vi "macro_LTV_DiffDriveCtrl_Traj_Sample_Execute.vi"() -> ()   [LabVIEW 2019, in "Trajectory_Library.lvlib"]
uses:
  Trajectory_Library.lvlib
  TypeDef/POSE2D.ctl
  TypeDef/TRANSLATION2D.ctl
  TypeDef/ROTATION2D.ctl
  TypeDef/TRAJ_STATE.ctl
  Enum/DCMOTOR_TYPES_ENUM.ctl
  Enum/DIFF_DRIVE_ToughBoxMini_GearChoice_ENUM.ctl
  LinearSystemId_CreateDriveTrainVelocitySystem.vi
  DCMotor_PickMotor_OLD.vi
  LinearSystem_New.vi
  MatBuilder_Create.vi
  MatBuilder_Fill.vi
  MatrixHelper_Zero.vi
  DCMotor_GetCIM.vi
  DCMotor_GetAndymark9015.vi
  DCMotor_GetAndymarkRs775_125.vi
  DCMotor_GetBag.vi
  DCMotor_GetBanebotsRs550.vi
  DCMotor_GetBanebotsRs775.vi
  DCMotor_GetFalcon500.vi
  DCMotor_GetMiniCIM.vi
  DCMotor_GetNEO.vi
  DCMotor_GetNEO550.vi
  DCMotor_GetRomiBuiltIn.vi
  DCMotor_GetVex775Pro.vi
  VI/DCMotor_GetAndymarkAM2235A.vi
  VI/DCMotor_GetAndymarkAM3493.vi
  MatrixHelper_CoerceSize.vi
  DCMotor_New.vi
  VI/Units_RotationsPerMinuteToRadiansPerSecond.vi
panel:
  in  "TRAJ_STATE":T1={"TimeSeconds"=0.0, "Velocity"=0.0, "Acceleration"=0.0, "POSE"={"TRANSLATION"={"X"=0.0, "Y"=0.0}, "ROTATION"={"VALUE"=0.0, "COS"=1.0, "SIN"=0.0}}, "Curvature"=0.0} {"POSE"."ROTATION"."SIN" format="%13.4f"; "POSE"."ROTATION"."COS" format="%13.4f"; "POSE"."ROTATION"."VALUE" format="%13.4f"; "POSE"."TRANSLATION"."Y" format="%14.3f"; "POSE"."TRANSLATION"."X" format="%14.3f"}
  in  "Right Velocity":dbl
  in  "Left Velocity":dbl
  out "Right Motor Dmd":dbl
  out "Left Motor Dmd":dbl
  in  "CurrentPose":T2={"TRANSLATION"={"X"=0.0, "Y"=0.0}, "ROTATION"={"VALUE"=0.0, "COS"=1.0, "SIN"=0.0}} {"ROTATION"."SIN" format="%13.4f"; "ROTATION"."COS" format="%13.4f"; "ROTATION"."VALUE" format="%13.4f"; "TRANSLATION"."Y" format="%14.3f"; "TRANSLATION"."X" format="%14.3f"}
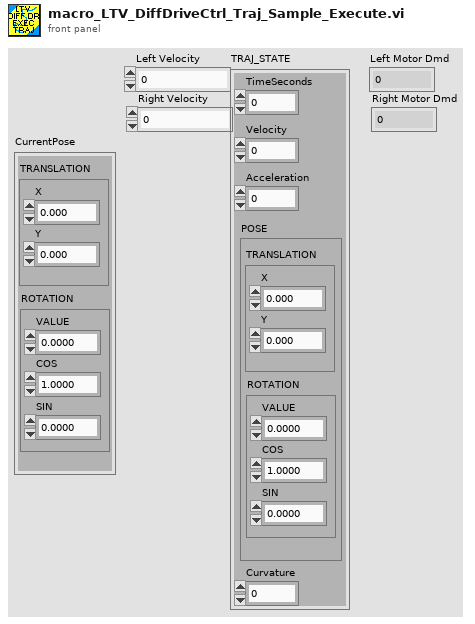
[diagram p1: front panel]
types:
  T1 = typedef "Trajectory_Library.lvlib/TRAJ_STATE.ctl" = cluster{"TimeSeconds":dbl, "Velocity":dbl, "Acceleration":dbl, "POSE":T2, "Curvature":dbl}
  T2 = typedef "Trajectory_Library.lvlib/POSE2D.ctl" = cluster{"TRANSLATION":T3, "ROTATION":T4}
  T3 = typedef "Trajectory_Library.lvlib/TRANSLATION2D.ctl" = cluster{"X":dbl, "Y":dbl}
  T4 = typedef "Trajectory_Library.lvlib/ROTATION2D.ctl" = cluster{"VALUE":dbl, "COS":dbl, "SIN":dbl}
  T5 = typedef "Trajectory_Library.lvlib/DIFF_DRIVE_ToughBoxMini_GearChoice_ENUM.ctl" = enum16{"Ratio_12_75", "Ratio_10_71", "Ratio_8_45", "Ratio_7_31", "Ratio_5_95"}
  T6 = typedef "Trajectory_Library.lvlib/DCMOTOR_TYPES_ENUM.ctl" = enum16{"CIM", "AndyMark 9015", "Andy Mark RS 775 125", "Bag", "BaneBots RS 550", "BaneBots RS 775", "Falcon 500", "Mini CIM", "NEO", "NEO 550", "Romi BuiltIn", "Vex 775 Pro", "Snow Blower AM 2235A", "Bosch Seat AM 3493"}
  T7 = typedef "Trajectory_Library.lvlib/LINEAR_SYSTEM.ctl" = cluster{"m_A":T8, "m_B":T8, "m_C":T8, "m_D":T8, "States":i32, "Inputs":i32, "Outputs":i32}
  T8 = typedef "NI_Matrix.lvlib/RealMatrix.ctl" = dbl[][]
  T9 = typedef "Trajectory_Library.lvlib/LTV_DIFF_DRIVE_CTRL_TOLERANCE.CTL" = cluster{"Max Heading Tolerance Rad":dbl, "Max X Tolerance M":dbl, "Max Y Tolerance M":dbl, "Max Left Vel Tol M/S":dbl, "Max Right Vel Tol M/S":dbl}
  T10 = typedef "Trajectory_Library.lvlib/LTV_DIFF_DRIVE_CTRL_CONTROL_PARAMS.CTL" = cluster{"Max left vel ctrl effort V":dbl, "Desired Heading Ctrl Tol Rad":dbl, "Desired Y Pos Meas Tol M":dbl, "Desired X Pos Ctrl Tol M":dbl, "Desired Left Vel Ctrl Tol M/S":dbl, "Desired Right Vel Ctrl Tol M/S":dbl, "Max right vel ctrl effort V":dbl}
  T11 = typedef "Trajectory_Library.lvlib/LTV_DIFF_DRIVE_CTRL_MODEL_PARAMS.CTL" = cluster{"Track Width":dbl, "Diff_Drive_Linear_System":T7, "LTV_DiffDriveCtrl_Control":T10, "LTV_DiffDriveCtrl_Tolerance":T9, "dT Sec":dbl}
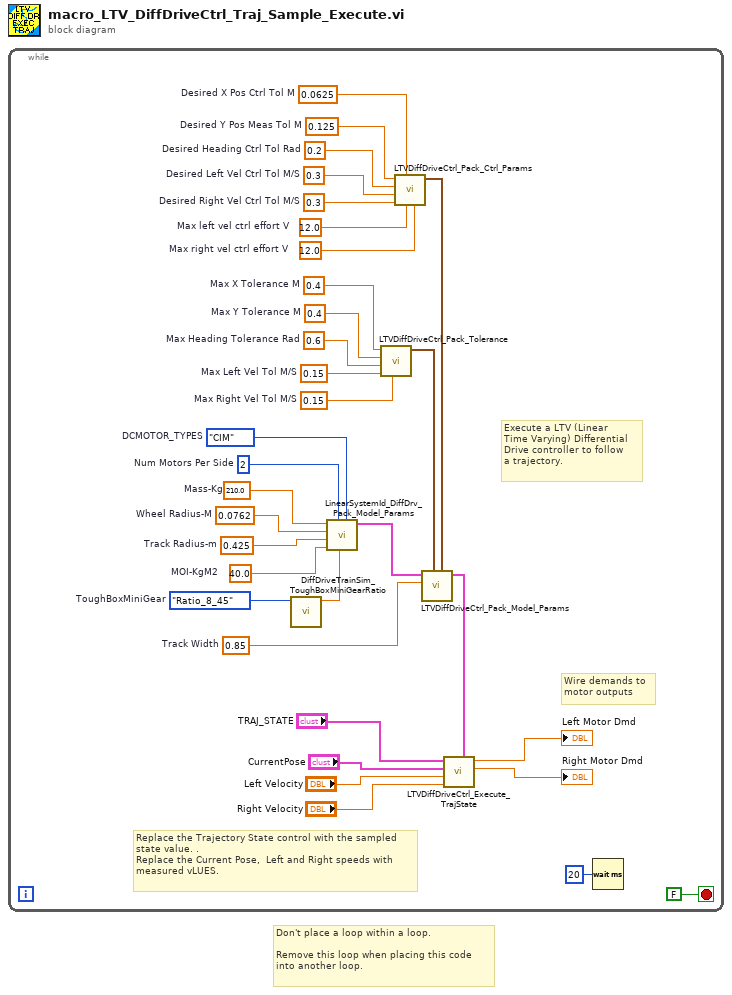
[diagram p0: block diagram]
diagram:
  # "Don't place a loop within a loop.\n \nRemove this loop when placing this code\ninto another loop."
  n1 = while {
    stop <- FALSE stop-if-true
    w6 = DIFF_DRIVE_ToughBoxMini_GearChoice_ENUM."Ratio_8_45"  # ToughBoxMiniGear
    w7 = 210.0  # Mass-Kg
    w8 = 0.0762  # Wheel Radius-M
    w9 = 0.425  # Track Radius-m
    w10 = 40.0  # MOI-KgM2
    w11 = 2  # Num Motors Per Side
    w12 = DCMOTOR_TYPES_ENUM."CIM"  # DCMOTOR_TYPES
    w14 = 0.4  # Max X Tolerance M
    w15 = 0.4  # Max Y Tolerance M
    w16 = 0.6  # Max Heading Tolerance Rad
    w17 = 0.15  # Max Left Vel Tol M/S
    w18 = 0.15  # Max Right Vel Tol M/S
    w19 = 0.125  # Desired Y Pos Meas Tol M
    w20 = 0.2  # Desired Heading Ctrl Tol Rad
    w21 = 0.3  # Desired Left Vel Ctrl Tol M/S
    w22 = 0.3  # Desired Right Vel Ctrl Tol M/S
    w23 = 0.0625  # Desired X Pos Ctrl Tol M
    w24 = 12.0  # Max left vel ctrl effort V
    w25 = 12.0  # Max right vel ctrl effort V
    w28 = 0.85  # Track Width
    # "Wire demands to\nmotor outputs"
    # "Replace the Trajectory State control with the sampled\nstate value. .\nReplace the Current Pose,  Left and Right speeds with\nmeasured vLUES."
    # "Execute a LTV (Linear \nTime Varying) Differential \nDrive controller to follow\na trajectory."
    n2 = call "DiffDriveTrainSim_ToughBoxMiniGearRatio.vi"("ToughBoxMiniGear"=w6) -> ("GearRatio"=w5:dbl)  [unwired: 10 in]
    n3 = call "LinearSystemId_DiffDrv_Pack_Model_Params.vi"("DCMOTOR_TYPES"=w12, "Gear Ratio"=w5, "Num Motors Per Side"=w11, "MOI-KgM2"=w10, "Track Radius-m"=w9, "Wheel Radius-M"=w8, "Mass-Kg"=w7) -> ("DiffDrv_LinearSystem"=w13:T7)  [unwired: 4 in]
    n4 = call "LTVDiffDriveCtrl_Pack_Tolerance.vi"("Max Right Vel Tol M/S"=w18, "Max Left Vel Tol M/S"=w17, "Max Heading Tolerance Rad"=w16, "Max Y Tolerance M"=w15, "Max X Tolerance M"=w14) -> ("LTV_DiffDriveCtrl_Tolerance"=w29:T9)  [unwired: 6 in]
    n5 = call "LTVDiffDriveCtrl_Pack_Ctrl_Params.vi"("Max right vel ctrl effort V"=w25, "Max left vel ctrl effort V"=w24, "Desired X Pos Ctrl Tol M"=w23, "Desired Right Vel Ctrl Tol M/S"=w22, "Desired Left Vel Ctrl Tol M/S"=w21, "Desired Heading Ctrl Tol Rad"=w20, "Desired Y Pos Meas Tol M"=w19) -> ("LTV_DiffDriveCtrl_Control"=w30:T10)  [unwired: 4 in]
    n6 = call "LTVDiffDriveCtrl_Pack_Model_Params.vi"("LTV_DiffDriveCtrl_Control"=w30, "LTV_DiffDriveCtrl_Tolerance"=w29, "Track Width"=w28, "Diff_Drive_Linear_System"=w13) -> ("LTV_DiffDriveCtrl_Model"=w31:T11)  [unwired: 7 in]
    n7 = call "LTVDiffDriveCtrl_Execute_TrajState.vi"("LTV_DiffDriveCtrl_Model"=w31, "Right Velocity"="Right Velocity", "Left Velocity"="Left Velocity", "CurrentPose"="CurrentPose", "TRAJ_STATE"="TRAJ_STATE") -> ("Right Motor Dmd"=→"Right Motor Dmd":dbl, "Left Motor Dmd"=→"Left Motor Dmd":dbl)  [unwired: 2 in, 3 out]
    n8 = Wait (ms)(milliseconds to wait=u32 20) -> ()  [unwired: 1 out]
  }
